vi "Add to Parent Priv.vi"(8 "Error In":errorcluster, 9 "Unique ID":string, 10 "Parent ID":string, 11 "Tree Dictionary":variant) -> (0 "Error Out":errorcluster, 3 "Tree Dictionary Out":variant)   [LabVIEW 2016, in "Tree Manager.lvclass"]
uses:
  Tree Manager.lvclass
  Typedefs/Tree.ctl
  <vilib>/Utility/error.llb/Error Cluster From Error Code.vi
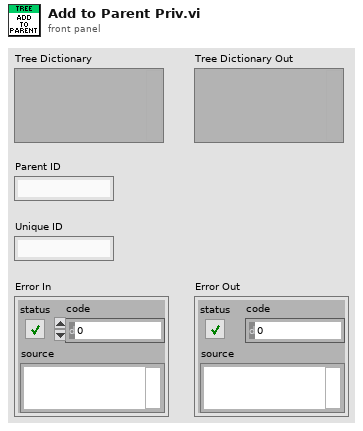
[diagram p1: front panel]
types:
  T1 = typedef "Tree Manager.lvclass/Tree.ctl" = cluster{"Unique ID":string, "Parent ID":string, "Child IDs":string[], "Data":variant, "Name":string}
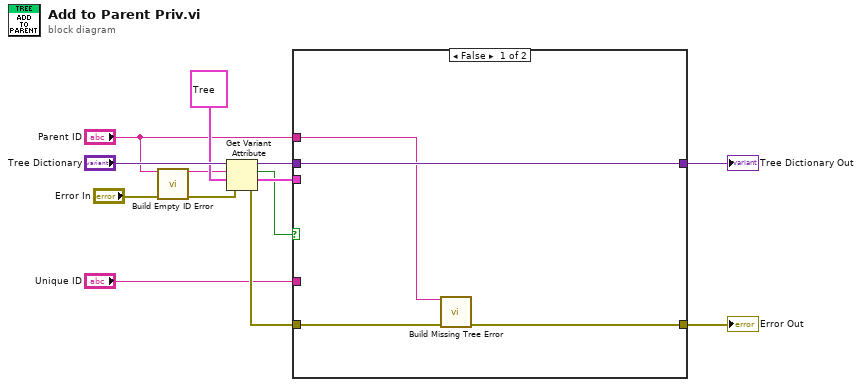
[diagram p0: block diagram]
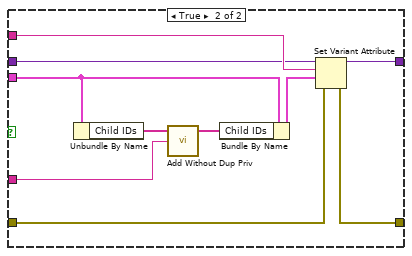
[diagram p2: hidden frame]
diagram:
  n1 = call "Build Empty ID Error.vi"("Unique ID"="Parent ID", "Error In"="Error In") -> ("Unique ID Out"=w2:string, "Error Out"=w1:errorcluster)  [unwired: 12 in]
  n2 = Get Variant Attribute(Variant="Tree Dictionary", name=w2, default value (empty Variant)=T1 {"Unique ID"="", "Parent ID"="", "Child IDs"=[], "Data"=variant, "Name"=""} ("Cluster of class private data"), error in=w1) -> (duplicate Variant=w10:variant, found=w6:bool, value=w9:T1, error out=w11:errorcluster)
  n3 = case shown="False" w6 {
    tunnel: [w17 w27] -> w13
    tunnel: [w14 w26] -> w12
    tunnel: w11 -> [w15 w25]
    tunnel: "Parent ID" -> [w16 w24]
    tunnel: w10 -> [w17 w22]
    tunnel: w9 -> [_ w21]
    tunnel: "Unique ID" -> [_ w19]
    frame False {
      n4 = call "Build Missing Tree Error.vi"("Unique ID"=w16, "Error In"=w15) -> ("Error Out"=w14:errorcluster)  [unwired: 13 in]
    }
    frame True {
      n5 = Unbundle By Name(w21) -> ("Child IDs"=w20:string[])
      n6 = call "Add Without Dup Priv.vi"("Unique ID"=w19, "Child IDs In"=w20) -> ("Child IDs Out"=w18:string[])  [unwired: 3 in]
      n7 = Bundle By Name(cluster=w21, "Child IDs"=w18) -> (w23:T1)
      n8 = Set Variant Attribute(Variant=w22, name=w24, value=w23, error in=w25) -> (Variant out=w27:variant, error out=w26:errorcluster)  [unwired: 1 out]
    }
  }
  "Tree Dictionary Out" <- w13
  "Error Out" <- w12
